vi "Interface.Get Error Queue.vi"(11 "Interface in":refnum<class "Interface.lvclass">) -> (2 "Error Queue":T1, 3 "Interface out":refnum<class "Interface.lvclass">)   [LabVIEW 2017, in "DSF.Engine.lvlib" / "Interface.lvclass"]
uses:
  Interface.lvclass
  Interface.Error Queue.Ref.ctl
  Interface.lvclass/Interface.ctl
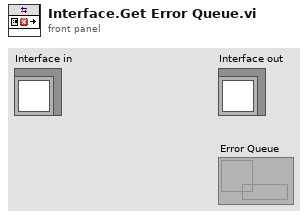
[diagram p1: front panel]
types:
  T1 = typedef "DSF.Engine.lvlib/Interface.lvclass/Interface.Error Queue.Ref.ctl" = refnum<queue>
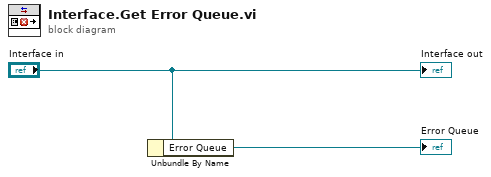
[diagram p0: block diagram]
diagram:
  n1 = Unbundle By Name("Interface in") -> ("Error Queue"=→"Error Queue":T1)
  "Interface out" <- "Interface in"
